vi "execution class name.vi"(8 "error in":errorcluster, 11 "shared memory module configuration":refnum<class "Shared Memory Configuration.lvclass">) -> (0 "error out":errorcluster, 2 "class name":string, 3 "shared memory module configuration out":refnum<class "Shared Memory Configuration.lvclass">)   [LabVIEW 2013, in "Shared Memory Configuration.lvclass"]
doc: "Provides an interface for determining the module runtime class associated with this module configuration. This class name can then be used to dynamically load or locate the runtime class for initialization purposes.Copyright 2016 National Instruments Corporation\n\nLicensed under the Apache License, Version 2.0 (the \"License\"); you may not use this file except in compliance with the License. You may obtain a copy of the License at http://www.apache.org/licenses/LICENSE-2.0\nUnless required by applicable law or agreed to in writing, software distributed under the License is distributed on an \"AS IS\" BASIS, WITHOUT WARRANTIES OR CONDITIONS OF ANY KIND, either express or implied. See the License for the specific language governing permissions and limitations under the License."
uses:
  Shared Memory Configuration.lvclass
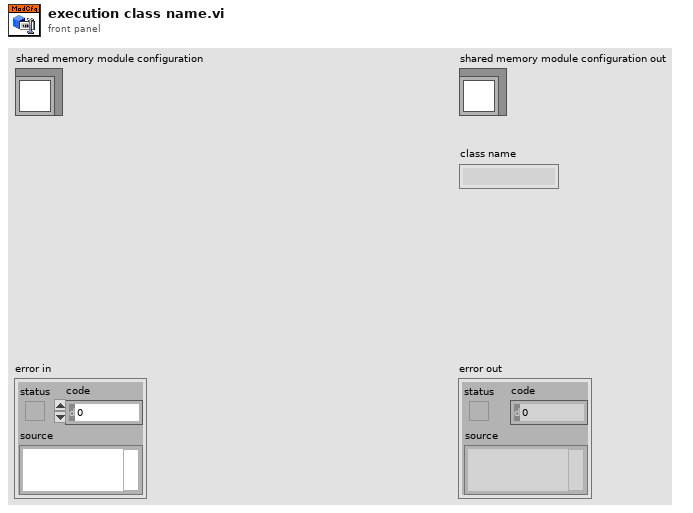
[diagram p1: front panel]
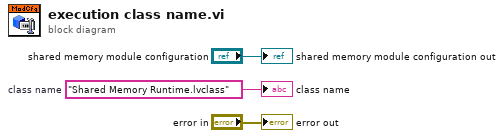
[diagram p0: block diagram]
diagram:
  w1 = "Shared Memory Runtime.lvclass"  # class name
  "error out" <- "error in"
  "shared memory module configuration out" <- "shared memory module configuration"
  "class name" <- w1
